vi "PicoScope6000ExampleRapidBlock.vi"() -> ()   [LabVIEW 2010]
uses:
  shared/PicoBuffers.ctl
  shared/Buffer and Transfer Settings.ctl
  shared/Acquisition Settings.ctl
  shared/Segment Range.ctl
  PicoScope6000Lib/PicoScope6000AnalogChannelSettings.ctl
panel:
  out "OverFlow":i16[](array[numeric]) format="%4b"
  out "Properties Panel":T1 {"Max Total Capture Time Available (sec)" format="%.3p"; "Sample Frequency" format="%.3p"; "Sample Internal" format="%.3p"; "Max Samples Available" format="%.3p"; "Total Capture Time (sec)" format="%.3p"}
  in  "Trigger Settings":T2={"Trigger Enabled"=TRUE, "Trigger Source"=enum."Channel A", "Trigger Threshold (Volts)"=0.0, "Trigger Direction"=2, "Trigger Delay (samples)"=0, "Auto Trigger Time (ms)"=1000} {"Trigger Direction" items=["Rising"=2, "Falling"=3]}
  in  "Channel A Settings":T3={"Enabled"=TRUE, "Coupling"=1, "Range"=6, "Analogue Offset"=0.0, "Bandwidth"=0} {"Bandwidth" items=["Full", "20 MHz"]; "Range" items=["10 mV", "20 mV", "50 mV", "100 mV", "200 mV", "500 mV", "1 V", "2 V", "5 V", "10 V", "20 V", "50 V ", "100 V"]; "Coupling" items=["AC", "DC 1 MOhm", "DC 50 Ohm"]}
  in  "Write ChA to file":bool
  in  "Stop Display":bool
  out "Capture Complete":bool
  in  "Run":bool
  in  "Display Buffer Index":i32
  in  "Segment Range":T4={"fromSegmentIndex"=0, "toSegmentIndex"=9} {"toSegmentIndex" format="%.4p"; "fromSegmentIndex" format="%.4p"}
  in  "nSegments":u64=10 format="%.4p"
  out "error out":errorcluster
  in  "Data file":path=path "PicoScopeospaExampleRapidBlock ChA Data"
  in  "Buffer and Transfer Settings":T5={"startIndex"=0, "Samples"=10000000, "Down Sample Ratio"=1, "Down-Sample Mode"=0} {"Down-Sample Mode" items=["None"=0, "Aggregate"=1, "Decimate"=2, "Average"=4]; "Down Sample Ratio" step=1; "Samples" format="%_6p"}
  in  "Acquisition Settings":T6={"preTriggerSamples"=0, "postTriggerSamples"=10000000, "timebase"=5} {"postTriggerSamples" format="%_6p"; "preTriggerSamples" format="%_6p"}
  in  "stop":bool
  out "Analog Channels":cluster{i32, sgl, "Data":dbl[]}[](graph)
  in  "Serial Number":string
  in  "Use Serial Number":bool
  in  "error in (no error)":errorcluster
  # "Bit 0 = ChA"
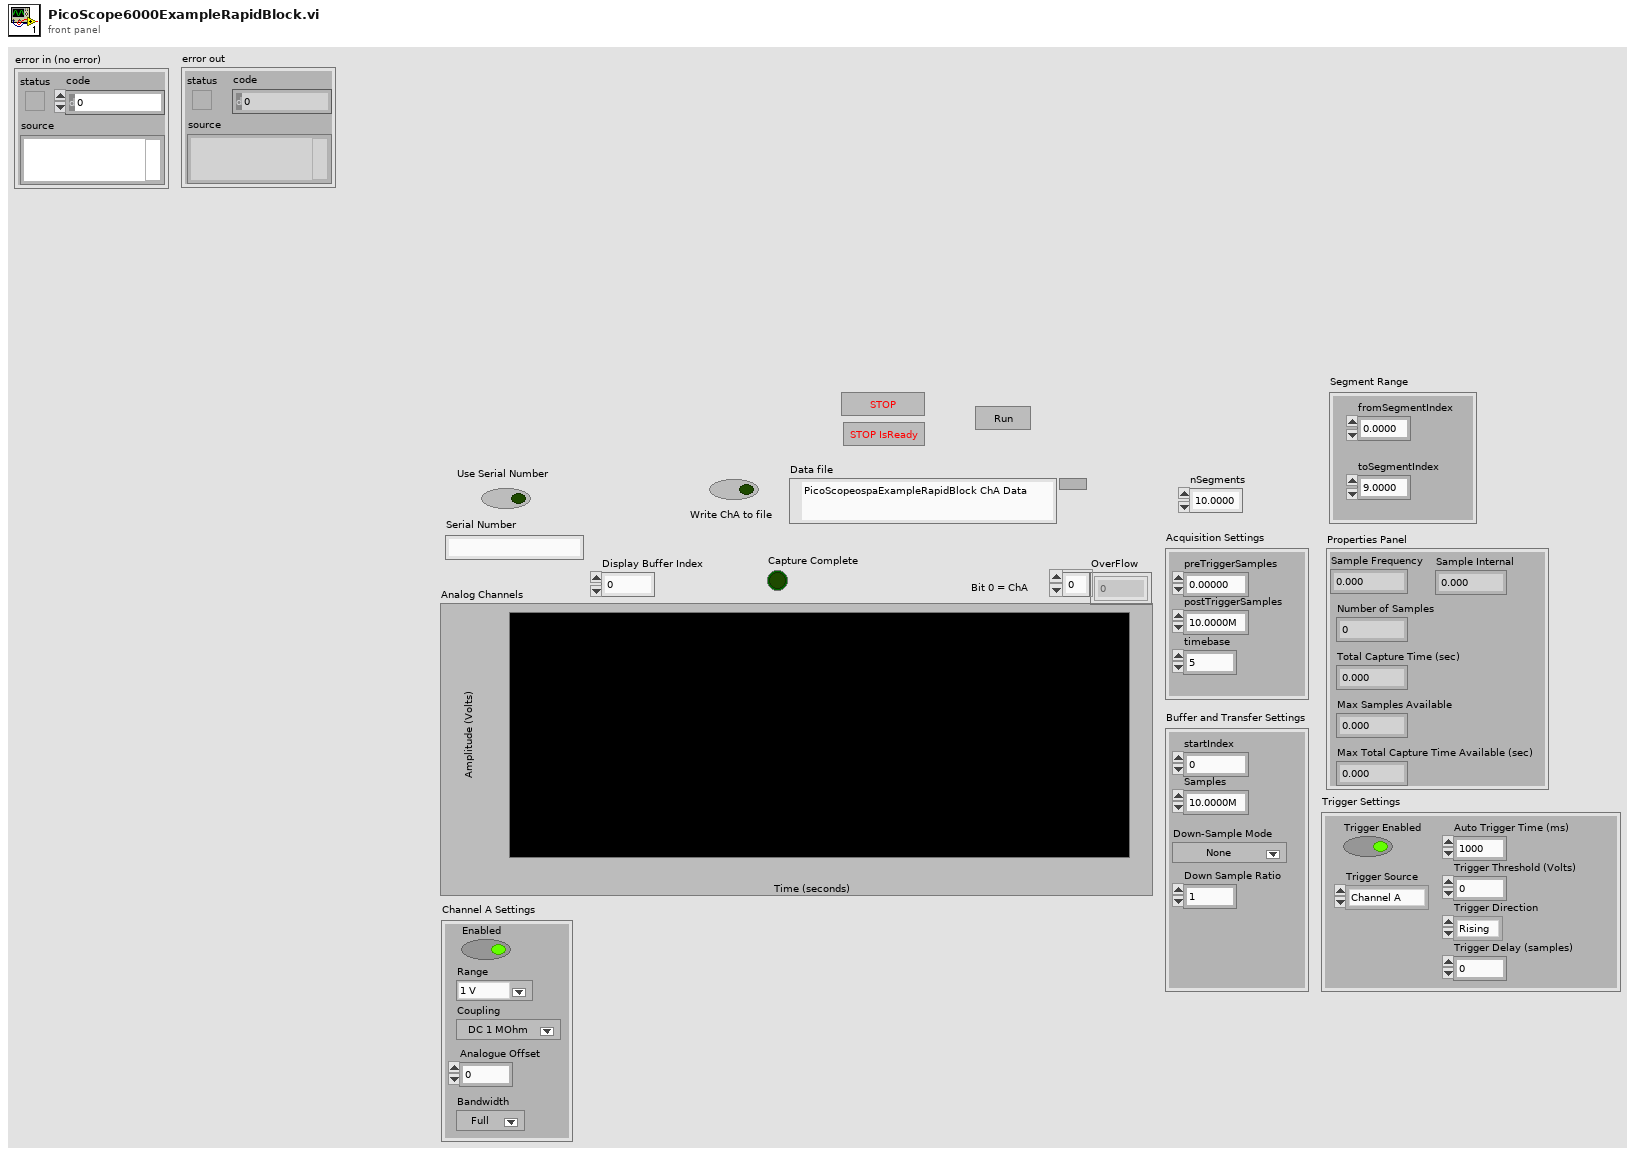
[diagram p1: front panel]
types:
  T1 = cluster{"Sample Frequency":sgl, "Sample Internal":sgl, "maxSamples":u32, "Number of Samples":u32, "Total Capture Time (sec) ":sgl, "Max Total Capture Time Available (sec)":sgl}
  T2 = cluster{"Trigger Enabled":bool, "Trigger Source":enum32{"Channel A", "Channel B", "Channel C", "Channel D", "External", "Aux."}, "Trigger Threshold (Volts)":dbl, "Trigger Direction":u16, "Trigger Delay (samples)":u32, "Auto Trigger Time (ms)":i16}
  T3 = typedef "PicoScope6000AnalogChannelSettings.ctl" = cluster{"Enabled":bool, "Coupling":u32, "Range":u32, "Analogue Offset":sgl, "Bandwidth":u32}
  T4 = typedef "Segment Range.ctl" = cluster{"fromSegmentIndex":u64, "toSegmentIndex":u64}
  T5 = typedef "Buffer and Transfer Settings.ctl" = cluster{"startIndex":u64, "Samples":u64, "Down Sample Ratio":u64, "Down-Sample Mode":u32}
  T6 = typedef "Acquisition Settings.ctl" = cluster{"preTriggerSamples":u64, "postTriggerSamples":u64, "timebase":u32}
  T7 = typedef "PicoBuffers.ctl" = cluster{"Max Buffer Pointers":u64[][][], "Min Buffer Pointers":u64[][][], "StreamingDataInfo":cluster{"Channel":u32, "Down-Sample Mode":u32, "PICO_DATA_TYPE":enum32{"PICO_INT8_T", "PICO_INT16_T", "PICO_INT32_T", "PICO_UINT32_T", "PICO_INT64_T", ""}, "Samples":i32, "bufferIndex":u64, "startIndex":i32, "overflow":i16}[][]}
  T8 = enum16{"open", "open or create", "create or replace", "create", "open (read-only)"}
  T9 = cluster{"Driver Version":string, "USB Version":string, "Hardware":string, "Variant":string, "Batch and Serial":string, "Cal Date":string, "Kernel Version":string, "Digital HW Version":string, "Analogue HW Version":string, "Firmware v1":string, "Firmware v2":string, "Channels":i16}
  T10 = cluster{"Channel A Buffer":i16[], "Channel B Buffer":i16[], "Channel C Buffer":i16[], "Channel D Buffer":i16[], "Channel E Buffer":i16[], "Channel F Buffer":i16[], "Channel G Buffer":i16[], "Channel H Buffer":i16[], "Port 0 Buffer":i16[], "Port 1 Buffer":i16[]}[]
  T11 = cluster{"Channel A Buffer":i16[], "Channel B Buffer":i16[], "Channel C Buffer":i16[], "Channel D Buffer":i16[], "Channel E Buffer":i16[], "Channel F Buffer":i16[], "Channel G Buffer":i16[], "Channel H Buffer":i16[], "Port 0 Buffer":i16[], "Port 1 Buffer":i16[]}
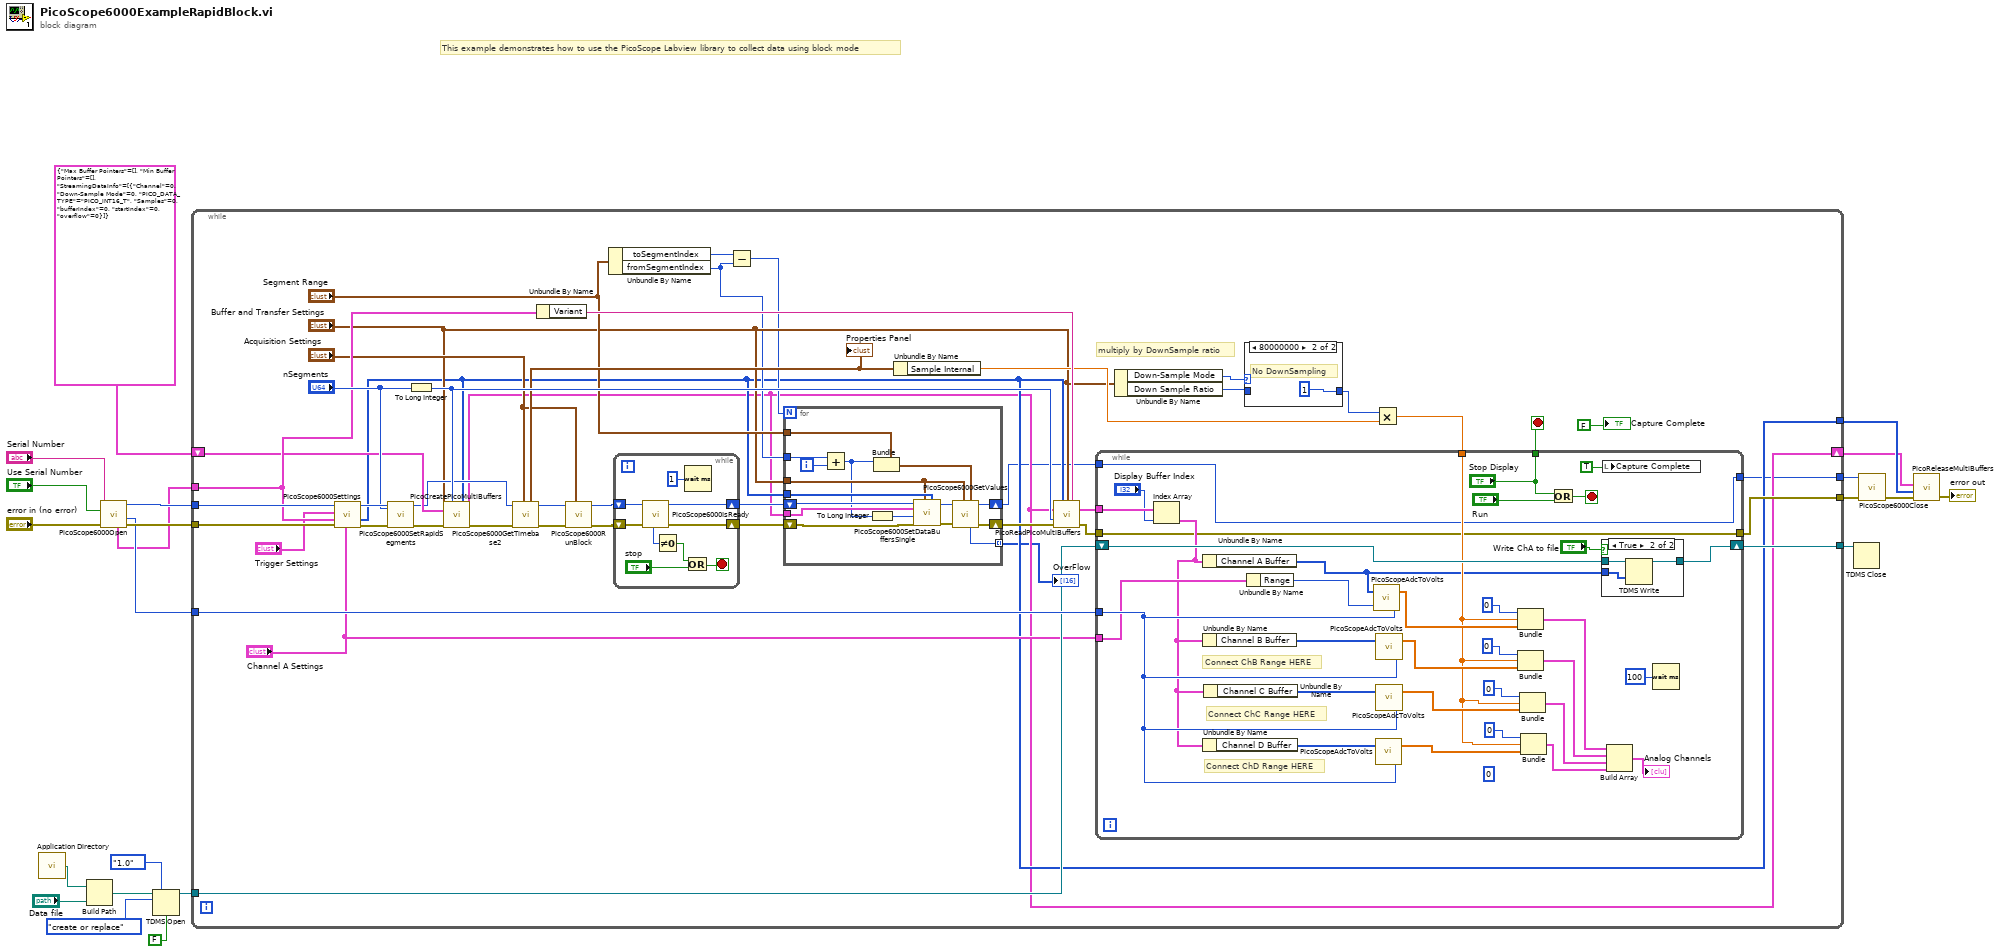
[diagram p0: block diagram]
diagram:
  # "This example demonstrates how to use the PicoScope Labview library to collect data using block mode"
  n1 = call <vilib>:"Application Directory.vi"() -> ("Application Directory"=w8:path)
  n2 = Build Path(base path=w8, name or relative path="Data file") -> (appended path=w9:path)
  n3 = call "PicoScope6000Open.vi"("error in (no error)"="error in (no error)", "Serial Number"="Serial Number", "Use Serial Number"="Use Serial Number") -> ("error out"=w18:errorcluster, "Max Adc value"=w17:i16, "handle"=w19:i16, "Device Info"=w4:T9)  [unwired: 4 in, 1 out]
  n4 = TDMS Open(6:FALSE ("disable buffering? (T)"), 7:enum16{"1.0", "2.0"}."1.0" ("file format version (2.0)"), 10:T8."create or replace" ("operation (0:open)"), 11:w9) -> (3:w6:refnum<k34>)  [unwired: 2 in, 1 out]
  n5 = while {
    tunnel: w4 -> [w42]
    tunnel: w17 -> [w66]
    tunnel: w19 -> [w68]
    tunnel: w18 -> [w67]
    tunnel: [w37] -> w15
    tunnel: [w27] -> w16
    tunnel: [w65] -> w7
    tunnel: w6 -> [w64]
    shift-right: [w26] -> w2
    shift-left: T7 {"Max Buffer Pointers"=[], "Min Buffer Pointers"=[], "StreamingDataInfo"=[[{"Channel"=0, "Down-Sample Mode"=0, "PICO_DATA_TYPE"=enum."PICO_INT16_T", "Samples"=0, "bufferIndex"=0, "startIndex"=0, "overflow"=0}]]} ("Data Pointers") -> [w41]
    tunnel: [w25] -> w1
    stop <- w47 stop-if-true
    # "multiply by DownSample ratio"
    n6 = call "PicoScope6000Settings.vi"("Channel A Settings"="Channel A Settings", "error in"=w67, "Device Info"=w42, "Trigger Settings"="Trigger Settings", "handle in"=w68) -> ("error out"=w63:errorcluster, "Enabled array"=w27:i16[], "handle out"=w62:i16)  [unwired: 4 in]
    n7 = call "PicoScope6000SetRapidSegments.vi"("nSegments"="nSegments", "error in (no error)"=w63, "handle in"=w62) -> ("error out"=w61:errorcluster, "handle out"=w32:i16)  [unwired: 6 in, 1 out]
    n8 = To Long Integer(number="nSegments") -> (32bit integer=w59:i32)
    n9 = call "PicoCreatePicoMultiBuffers.vi"("Number of Buffers"=w59, "Buffer and Transfer Settings"="Buffer and Transfer Settings", "enabled array"=w27, "Data Pointers In"=w41, "error in (no error)"=w61) -> ("Data Pointers"=w26:T7, "error out"=w33:errorcluster)  [unwired: 9 in]
    n10 = call "PicoScope6000GetTimebase2.vi"("Acquisition Settings"="Acquisition Settings", "error in (no error)"=w33, "handle in"=w32) -> ("error out"=w51:errorcluster, "handle out"=w52:i16, "Properties Panel"=w55:T1)  [unwired: 6 in]
    "Properties Panel" <- w55
    n11 = Unbundle By Name(w42) -> ("Variant"=w45:string)
    n12 = call "PicoScope6000RunBlock.vi"("Acquisition Settings"="Acquisition Settings", "error in (no error)"=w51, "handle in"=w52) -> ("error out"=w50:errorcluster, "handle out"=w49:i16)  [unwired: 5 in, 2 out]
    n13 = Unbundle By Name("Segment Range") -> ("toSegmentIndex"=w44:u64, "fromSegmentIndex"=w29:u64)
    n14 = while {
      shift-right: [w130] -> w36
      shift-left: w50 -> [w131]
      shift-right: [w129] -> w34
      shift-left: w49 -> [w128]
      stop <- w126 stop-if-true
      n15 = call "PicoScope6000IsReady.vi"("error in (no error)"=w131, "handle in"=w128) -> ("error out"=w130:errorcluster, "handle out"=w129:i16, "ready"=w127:i16)  [unwired: 7 in]
      n16 = Not Equal To 0?(x=w127) -> (x != 0?=w125:bool)
      n17 = Or(x=w125, y="stop") -> (x .or. y?=w126:bool)
      n18 = Wait (ms)(milliseconds to wait=u32 1) -> ()  [unwired: 1 out]
    }
    n19 = Subtract(x=w44, y=w29) -> (x-y=w28:u64)
    n20 = for {
      N: w28 -> [_]
      shift-right: [w84] -> w24
      shift-left: w34 -> [w75]
      shift-right: [w83] -> w35
      shift-left: w36 -> [w76]
      tunnel: w29 -> [w70]
      tunnel: "Segment Range" -> [w81]
      tunnel: [w79] -> w23 mode=indexing
      tunnel: w26 -> [w74]
      tunnel: w27 -> [w73]
      tunnel: "Buffer and Transfer Settings" -> [w72]
      i -> [w82]
      n21 = Add(x=w70, y=w82) -> (x+y=w69:u64)
      n22 = To Long Integer(number=w69) -> (32bit integer=w71:i32)
      n23 = Bundle(cluster=w81, "fromSegmentIndex"=w69) -> (w80:T4)  [unwired: 1 in]
      n24 = call "PicoScope6000SetDataBuffersSingle.vi"("enabled array"=w73, "Buffer and Transfer Settings"=w72, "error in (no error)"=w76, "waveform"=w71, "Data Pointers In"=w74, "handle in"=w75) -> ("error out"=w78:errorcluster, "handle out"=w77:i16)  [unwired: 4 in]
      n25 = call "PicoScope6000GetValues.vi"("Segment Range"=w80, "Buffer and Transfer Settings"=w72, "error in (no error)"=w78, "handle in"=w77) -> ("error out"=w83:errorcluster, "handle out"=w84:i16, "overflow"=w79:i16)  [unwired: 4 in, 1 out]
    }
    "OverFlow" <- w23
    n26 = Unbundle By Name(w55) -> ("Sample Internal"=w38:sgl)
    n27 = call "PicoReadPicoMultiBuffers.vi"("enabled array"=w27, "Buffer and Transfer Settings"="Buffer and Transfer Settings", "Variant"=w45, "Data Pointers"=w26, "No of Buffers"=w59, "error in (no error)"=w35) -> ("MultiBuffers (Max or non-aggregated)"=w58:T10, "error out"=w48:errorcluster)  [unwired: 7 in, 1 out]
    n28 = Unbundle By Name("Buffer and Transfer Settings") -> ("Down-Sample Mode"=w56:u32, "Down Sample Ratio"=w57:u64)
    n29 = case shown="80000000" w56 {
      tunnel: [w132 u64 1 ("Down Sample Ratio")] -> w53
      tunnel: w57 -> [w132 _]
      frame Default {
      }
      frame -2147483648 {
        # "No DownSampling"
      }
    }
    n30 = Multiply(x=w53, y=w38) -> (x*y=w54:sgl)
    n31 = while {
      tunnel: w66 -> [w118]
      tunnel: "Channel A Settings" -> [w117]
      tunnel: w58 -> [w97]
      tunnel: w54 -> [w96]
      shift-right: [w116] -> w65
      shift-left: w64 -> [w115]
      tunnel: [w86] -> w37
      tunnel: w48 -> [w86]
      tunnel: ["Stop Display"] -> w47
      tunnel: [w85] -> w25
      tunnel: w24 -> [w85]
      stop <- w90 stop-if-true
      (unwired) 0
      # "Connect ChD Range HERE"
      # "Connect ChC Range HERE"
      # "Connect ChB Range HERE"
      n32 = Index Array(array=w97, index="Display Buffer Index") -> (element=w95:T11)
      n33 = Unbundle By Name(w95) -> ("Channel A Buffer"=w94:i16[])
      n34 = Unbundle By Name(w95) -> ("Channel B Buffer"=w111:i16[])
      n35 = Unbundle By Name(w95) -> ("Channel D Buffer"=w105:i16[])
      n36 = Unbundle By Name(w95) -> ("Channel C Buffer"=w106:i16[])
      n37 = Unbundle By Name(w117) -> ("Range"=w113:u32)
      n38 = call "PicoScopeAdcToVolts.vi"("Max_adc"=w118, "Range Index"=w113, "Data"=w94) -> ("Data"=w98:dbl[])
      n39 = call "PicoScopeAdcToVolts.vi"("Max_adc"=w118, "Data"=w105) -> ("Data"=w101:dbl[])  [unwired: 1 in]
      n40 = call "PicoScopeAdcToVolts.vi"("Max_adc"=w118, "Data"=w111) -> ("Data"=w110:dbl[])  [unwired: 1 in]
      n41 = call "PicoScopeAdcToVolts.vi"("Max_adc"=w118, "Data"=w106) -> ("Data"=w102:dbl[])  [unwired: 1 in]
      n42 = Bundle(0, w96, "Data"=w98) -> (w109:cluster{i32, sgl, "Data":dbl[]})  [unwired: 1 in]
      n43 = Bundle(0, w96, "Data"=w110) -> (w108:cluster{i32, sgl, "Data":dbl[]})  [unwired: 1 in]
      n44 = Bundle(0, w96, "Data"=w102) -> (w100:cluster{i32, sgl, "Data":dbl[]})  [unwired: 1 in]
      n45 = Bundle(0, w96, "Data"=w101) -> (w99:cluster{i32, sgl, "Data":dbl[]})  [unwired: 1 in]
      n46 = Or(x="Stop Display", y="Run") -> (x .or. y?=w90:bool)
      n47 = case shown="True" "Write ChA to file" {
        tunnel: [w119 w122] -> w116
        tunnel: w115 -> [w119 w121]
        tunnel: w94 -> [_ w120]
        frame False {
        }
        frame True {
          n48 = TDMS Write(0:w121, 9:w120) -> (4:w122:refnum<k34>)  [unwired: 4 in, 3 out]
        }
      }
      n49 = local write "Capture Complete"(TRUE ("Capture Complete")) -> ()
      n50 = Build Array(w109, w108, w100, w99) -> (→"Analog Channels":cluster{i32, sgl, "Data":dbl[]}[])
      n51 = Wait (ms)(milliseconds to wait=u32 100) -> ()  [unwired: 1 out]
    }
    "Capture Complete" <- FALSE ("Capture Complete")
  }
  n52 = TDMS Close(11:w7) -> ()  [unwired: 1 in, 2 out]
  n53 = call "PicoScope6000Close.vi"("error in (no error)"=w15, "handle"=w1) -> ("error out"=w14:errorcluster)  [unwired: 8 in, 1 out]
  n54 = call "PicoReleaseMultiBuffers.vi"("error in (no error)"=w14, "Enabled array"=w16, "Data Pointers"=w2) -> ("error out"=→"error out":errorcluster)  [unwired: 7 in, 1 out]
